vi "CDO to Channel Settings.vi"(8 "error in":errorcluster, 9 "channel default values":dbl[](array[numeric]), 10 "channel names":string[](array[string]), 11 "SD Module in":refnum<class "SD Module.lvclass">) -> (0 "error out":errorcluster, 2 "channel settings":T2[](array[typedef]), 3 "drive from slot":T1)   [LabVIEW 2017, in "Scan Engine Scripting.lvlib"]
uses:
  Scan Engine Scripting.lvlib
  Modules/Mode Classes/Controls/counter driven output channel settings.ctl
  Modules/Channel Classes/Counter Driven Output Channel/Counter Driven State.ctl
  Modules.lvlibp/SD Module/SD Module.lvclass
  Modules/Mode Classes/Counter Driven Output Mode/Drive from Slot.ctl
  Modules/Channel Classes/Counter Driven Output Channel/Counter Driven Output Channel.lvclass
  Modules/Mode Classes/Counter Driven Output Mode/Counter Driven Output Mode.lvclass
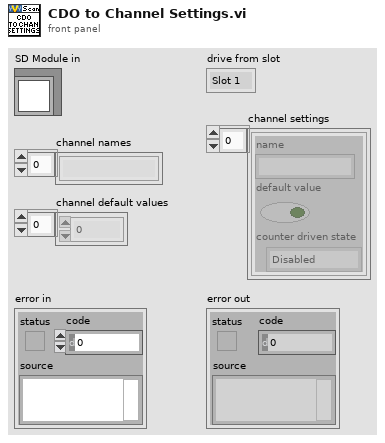
[diagram p1: front panel]
types:
  T1 = typedef "Scan Engine Scripting.lvlib/Counter Driven Output Mode.lvclass/Drive from Slot.ctl" = enum16{"Slot 1", "Slot 2", "Slot 3", "Slot 4", "Slot 5", "Slot 6", "Slot 7", "Slot 8"}
  T2 = typedef "Scan Engine Scripting.lvlib/counter driven output channel settings.ctl" = cluster{"name":string, "default value":bool, "counter driven state":T3}
  T3 = typedef "Scan Engine Scripting.lvlib/Counter Driven Output Channel.lvclass/Counter Driven State.ctl" = enum16{"Disabled", "Enabled"}
  T4 = typedef "Modules.lvlibp/SD Module.lvclass/CDO.ctl" = cluster{"Drive From Slot":u32, "CDO Channels":T5[]}
  T5 = typedef "Modules.lvlibp/SD Module.lvclass/CDO Channel.ctl" = cluster{"Counter driven enabled":bool}
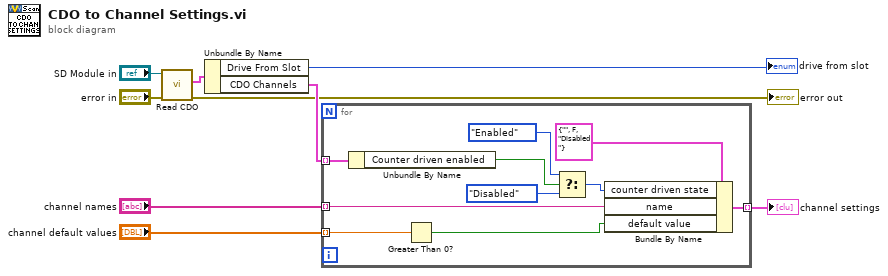
[diagram p0: block diagram]
diagram:
  n1 = call-dynamic "Read CDO.vi"("error in (no error)"="error in", "SD Module in"="SD Module in") -> ("error out"=→"error out":errorcluster, "CDO"=w4:T4)  [unwired: 7 in, 1 out]
  n2 = Unbundle By Name(w4) -> ("Drive From Slot"=→"drive from slot":u32, "CDO Channels"=w7:T5[])
  n3 = for {
    tunnel: w7 -> [w19] mode=indexing
    tunnel: [w17] -> w6 mode=indexing
    tunnel: "channel names" -> [w12] mode=indexing
    tunnel: "channel default values" -> [w11] mode=indexing
    n4 = Unbundle By Name(w19) -> ("Counter driven enabled"=w14:bool)
    n5 = Greater Than 0?(x=w11) -> (x > 0?=w10:bool)
    n6 = Select(t=Counter_Driven_State."Enabled" ("counter driven state"), s=w14, f=Counter_Driven_State."Disabled" ("counter driven state")) -> (s? t:f=w13:T3)
    n7 = Bundle By Name(cluster=T2 {"name"="", "default value"=FALSE, "counter driven state"=enum."Disabled"} ("channel settings"), "counter driven state"=w13, "name"=w12, "default value"=w10) -> (w17:T2)
  }
  "channel settings" <- w6
